vi "产生一维数组.vi"(11 "Numeric":i32) -> (3 "Array":i32[](array[numeric]))   [LabVIEW 2015]
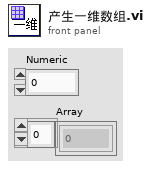
[diagram p1: front panel]
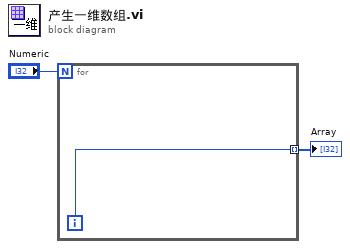
[diagram p0: block diagram]
diagram:
  n1 = for {
    N: "Numeric" -> [_]
    tunnel: [w3] -> w1 mode=indexing
    i -> [w3]
  }
  "Array" <- w1
